vi "WS1021 VSA Convert Data.vi"(0 "VSA_Cap(fF)":string[][](array[string]), 1 "Voltage(V)":string[][](array[string]), 11 "error in (no error)":errorcluster) -> (2 "BT_VSA_V1":string[][](array[string]), 3 "BT_VSA_V2":string[][](array[string]), 4 "BT_VSA_V3":string[][](array[string]), 10 "VSA_V3":string[][](array[string]), 13 "VSA_V1":string[][](array[string]), 14 "VSA_V2":string[][](array[string]), 15 "error out":errorcluster)   [LabVIEW 2017]
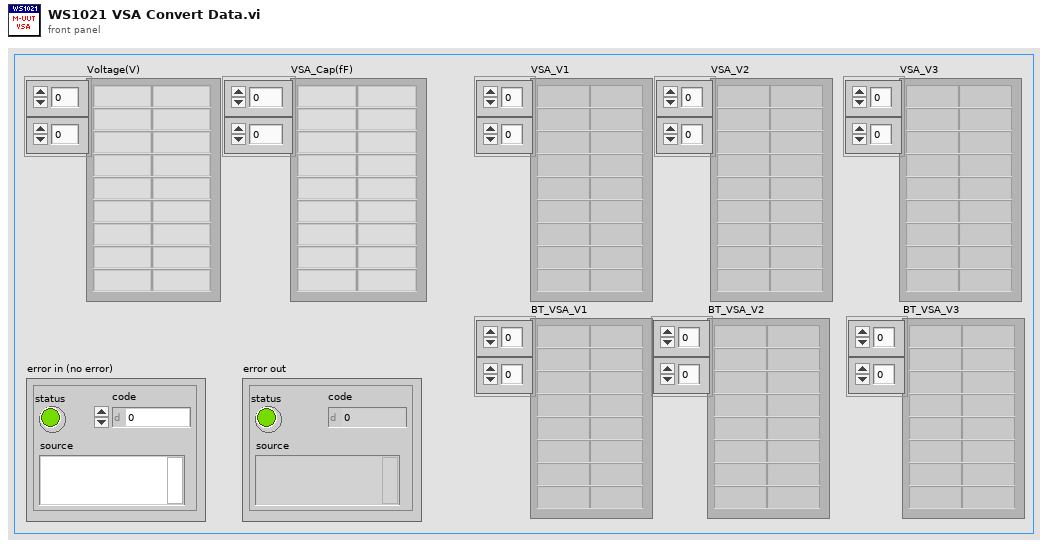
[diagram p1: front panel]
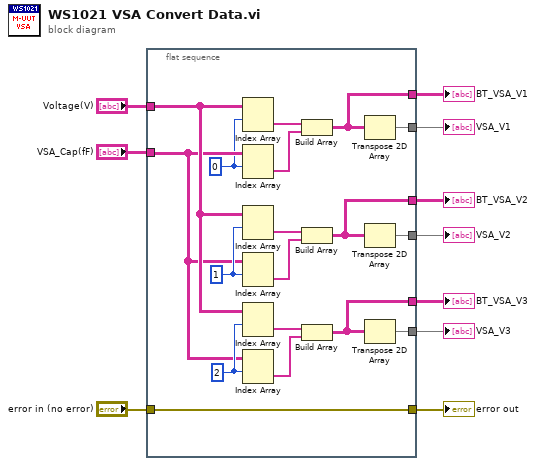
[diagram p0: block diagram]
diagram:
  n1 = flat-sequence {
    tunnel: "error in (no error)" -> [w22]
    tunnel: [w22] -> w9
    tunnel: "Voltage(V)" -> [w19]
    tunnel: "VSA_Cap(fF)" -> [w18]
    tunnel: [w17] -> w6
    tunnel: [w16] -> w5
    tunnel: [w15] -> w4
    tunnel: [w14] -> w1
    tunnel: [w13] -> w2
    tunnel: [w12] -> w3
    frame #0 {
      w20 = 2 ("disabled index (col)")
      w21 = 1 ("disabled index (col)")
      w11 = 0 ("disabled index (col)")
      n2 = Index Array(array=w19, index (row)=w11) -> (element=w28:string[])  [unwired: 1 in]
      n3 = Index Array(array=w18, index (row)=w11) -> (element=w27:string[])  [unwired: 1 in]
      n4 = Index Array(array=w19, index (row)=w21) -> (element=w25:string[])  [unwired: 1 in]
      n5 = Index Array(array=w18, index (row)=w21) -> (element=w26:string[])  [unwired: 1 in]
      n6 = Index Array(array=w19, index (row)=w20) -> (element=w24:string[])  [unwired: 1 in]
      n7 = Index Array(array=w18, index (row)=w20) -> (element=w23:string[])  [unwired: 1 in]
      n8 = Build Array(w28, w27) -> (w12:string[][])
      n9 = Build Array(w25, w26) -> (w13:string[][])
      n10 = Build Array(w24, w23) -> (w14:string[][])
      n11 = Transpose 2D Array(2D array=w12) -> (transposed array=w17:string[][])
      n12 = Transpose 2D Array(2D array=w13) -> (transposed array=w16:string[][])
      n13 = Transpose 2D Array(2D array=w14) -> (transposed array=w15:string[][])
    }
  }
  "error out" <- w9
  "VSA_V1" <- w6
  "VSA_V2" <- w5
  "VSA_V3" <- w4
  "BT_VSA_V1" <- w3
  "BT_VSA_V2" <- w2
  "BT_VSA_V3" <- w1
